vi "Typy_symul.vi"(8 "error in (no error)":errorcluster, 10 "Kanaly in":T1) -> (0 "error out":errorcluster, 2 "Kanaly out":T1)   [LabVIEW 2014]
doc: "Nadaje typ przebiegu, AI, DI, Zw"
uses:
  Kontrolki/Przetwarzanie/Kanaly.ctl
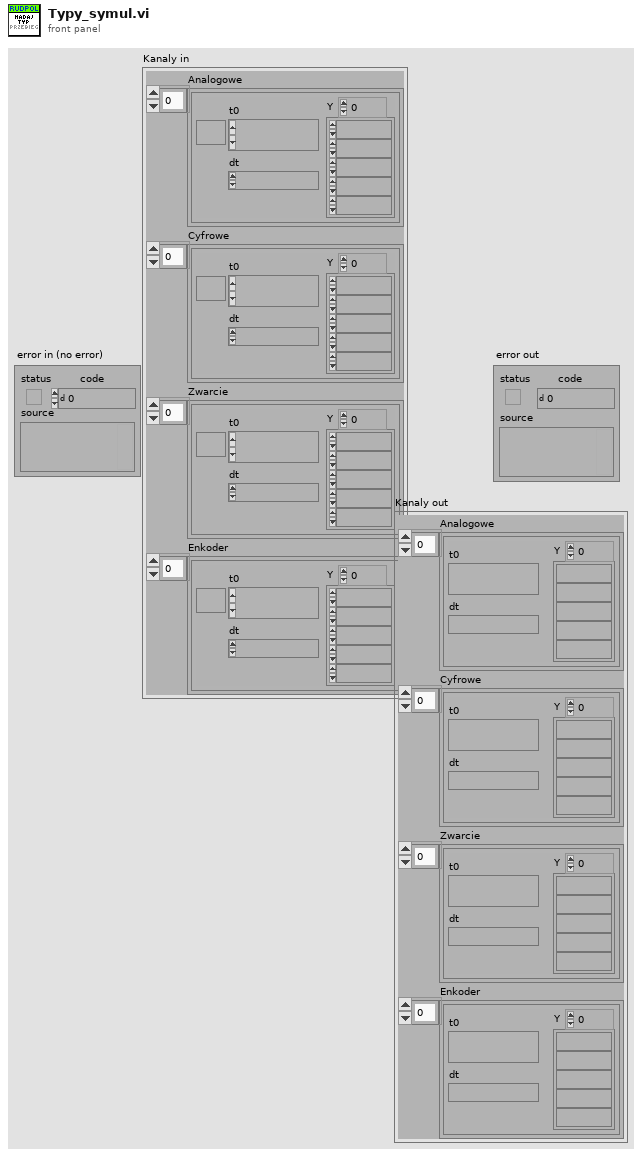
[diagram p1: front panel]
types:
  T1 = typedef "Kanaly.ctl" = cluster{"Analogowe":waveform(dbl)[], "Cyfrowe":waveform(dbl)[], "Zwarcie":waveform(dbl)[], "Enkoder":waveform(dbl)[]}
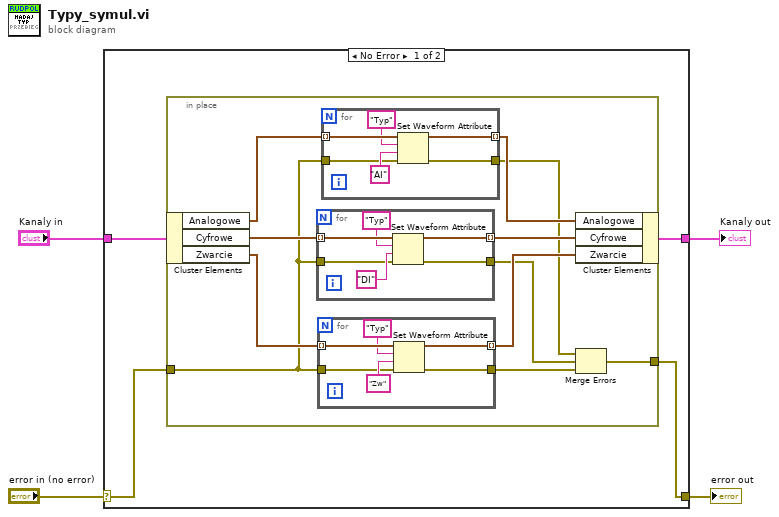
[diagram p0: block diagram]
diagram:
  n1 = case shown="No Error" "error in (no error)" {
    selector: "error in (no error)" -> [w6 w39]
    tunnel: [w5 w39] -> w3
    tunnel: "Kanaly in" -> [w8 w38]
    tunnel: [w7 w38] -> w1
    frame No Error {
      n2 = in-place {
        in-place-border: w6 -> [w13]
        in-place-border: [w11] -> w5
        n3 = in-place-cluster #1(w8) -> ("Analogowe"=w19:waveform(dbl)[], "Cyfrowe"=w17:waveform(dbl)[], "Zwarcie"=w15:waveform(dbl)[])
        n4 = for {
          tunnel: w17 -> [w31] mode=indexing
          tunnel: [w29] -> w16 mode=indexing
          tunnel: w13 -> [w27]
          tunnel: [w26] -> w10
          n5 = Set Waveform Attribute(4:w27, 5:"DI", 6:"Typ", 7:w31) -> (0:w26:errorcluster, 3:w29:waveform(dbl))  [unwired: 1 out]
        }
        n6 = for {
          tunnel: w15 -> [w25] mode=indexing
          tunnel: [w22] -> w14 mode=indexing
          tunnel: w13 -> [w21]
          tunnel: [w20] -> w12
          n7 = Set Waveform Attribute(4:w21, 5:"Zw", 6:"Typ", 7:w25) -> (0:w20:errorcluster, 3:w22:waveform(dbl))  [unwired: 1 out]
        }
        n8 = for {
          tunnel: w19 -> [w37] mode=indexing
          tunnel: [w34] -> w18 mode=indexing
          tunnel: w13 -> [w33]
          tunnel: [w32] -> w9
          n9 = Set Waveform Attribute(4:w33, 5:"AI", 6:"Typ", 7:w37) -> (0:w32:errorcluster, 3:w34:waveform(dbl))  [unwired: 1 out]
        }
        n10 = in-place-cluster #1("Analogowe"=w18, "Cyfrowe"=w16, "Zwarcie"=w14) -> (w7:T1)
        n11 = Merge Errors(w9, w10, w12) -> (w11:errorcluster)
      }
    }
    frame Error {
    }
  }
  "error out" <- w3
  "Kanaly out" <- w1
